vi "Write Receive Binary Data.vi"(8 "error in (no error)":errorcluster, 9 "values":u8[](array[numeric]), 10 "starting address":u16, 11 "standard data model in":refnum<class "WebSocket Data Model.lvclass">) -> (0 "error out":errorcluster, 3 "standard data model out":refnum<class "WebSocket Data Model.lvclass">)   [LabVIEW 2021, in "WebSockets.lvlib" / "WebSocket Data Model.lvclass"]
doc: "Writes the values of multiple input register values in series, starting at address M."
uses:
  WebSocket Data Model.lvclass
  WebSocket Data Model.lvclass/WebSocket Data Model.ctl
  WebSocket/Opcodes.ctl
  WebSocket/WebSocket.lvclass
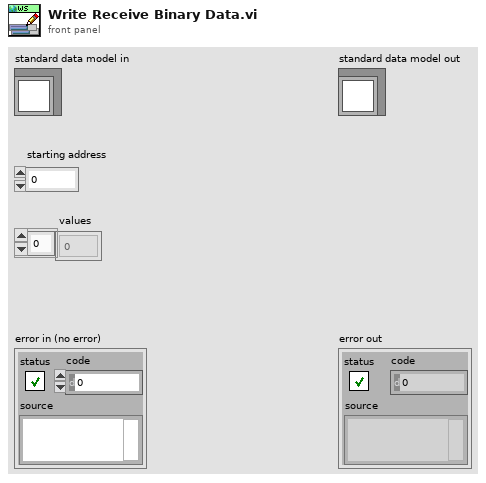
[diagram p1: front panel]
types:
  T1 = typedef "WebSockets.lvlib/WebSocket.lvclass/Opcodes.ctl" = u8
  T2 = typedef "WebSockets.lvlib/WebSocket Data Model.lvclass/Data Model.ctl" = cluster{"UTC":u64, "Receive Binary Data":u8[], "Receive Text Data":string, "Send Binary Data":u8[], "Send Text Data":string, "ES":u8}
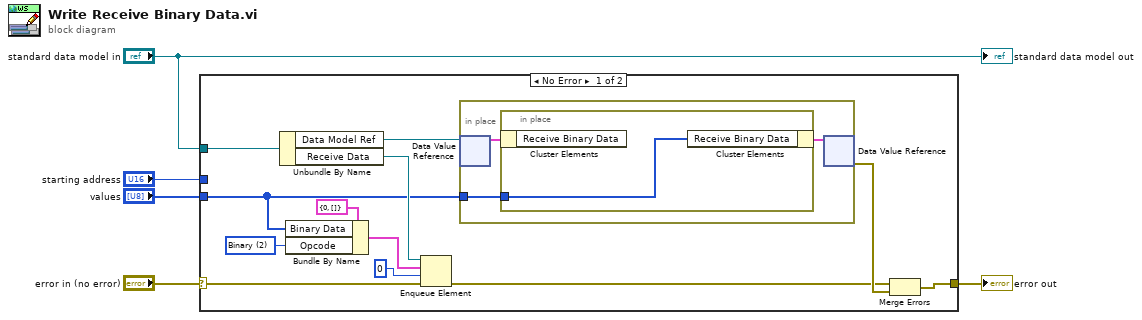
[diagram p0: block diagram]
diagram:
  n1 = case shown="No Error" "error in (no error)" {
    selector: "error in (no error)" -> [w13 w22]
    tunnel: "starting address" -> [_ _]
    tunnel: "values" -> [w8 _]
    tunnel: "standard data model in" -> [w10 _]
    tunnel: [w17 w22] -> w2
    frame No Error {
      w6 = T1 2 items=["Cont. Frame"=0, "Text"=1, "Binary"=2, "Close Frame"=8, "Ping"=9, "Pong"=10] ("Opcode")
      n2 = Unbundle By Name(w10) -> ("Data Model Ref"=w11:refnum<data-value>, "Receive Data"=w14:refnum<queue>)
      n3 = Bundle By Name(cluster=cluster{"Opcode":T1, "Binary Data":u8[]} {"Opcode"=0, "Binary Data"=[]} ("Data"), "Binary Data"=w8, "Opcode"=w6) -> (w7:cluster{"Opcode":T1, "Binary Data":u8[]})
      n4 = Enqueue Element(queue=w14, element=w7, timeout in ms (-1)=0, error in (no error)=w13) -> (error out=w12:errorcluster)  [unwired: 2 out]
      n5 = in-place {
        in-place-border: w8 -> [w20]
        n6 = in-place-dvr #1(w11) -> (w19:T2)  [unwired: 1 out]
        n7 = in-place {
          in-place-border: w20 -> [w21]
          n8 = in-place-cluster #2(w19) -> ()  [unwired: 1 out]
          n9 = in-place-cluster #2("Receive Binary Data"=w21) -> (w18:T2)
        }
        n10 = in-place-dvr #1(w18) -> (w16:errorcluster)  [unwired: 1 out]
      }
      n11 = Merge Errors(w12, w16) -> (w17:errorcluster)
    }
    frame Error {
    }
  }
  "error out" <- w2
  "standard data model out" <- "standard data model in"
